vi "testLeonardo.vi"() -> ()   [LabVIEW 2014]
panel:
  out "Buttons":bool[](array[boolean])
  in  "stop":bool
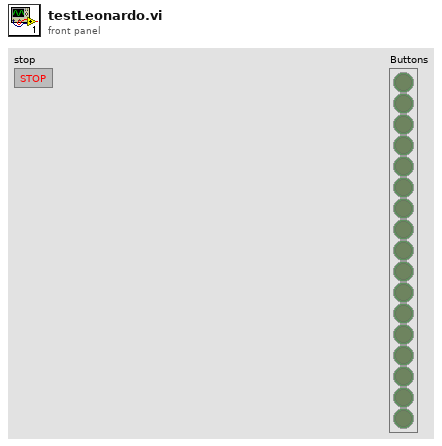
[diagram p1: front panel]
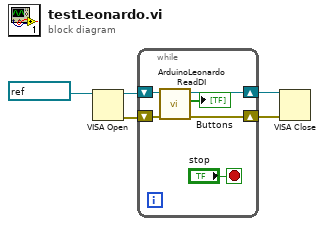
[diagram p0: block diagram]
diagram:
  n1 = VISA Open(VISA resource name=refnum<visa-resource-name> "COM4") -> (VISA resource name=w5:refnum<visa-resource-name>, error out=w1:errorcluster)  [unwired: 4 in]
  n2 = while {
    shift-right: [w9] -> w2
    shift-left: w5 -> [w11]
    shift-right: [w10] -> w3
    shift-left: w1 -> [w8]
    stop <- "stop" stop-if-true
    n3 = call "ArduinoLeonardoReadDI.vi"("error in (no error)"=w8, "VISA resource name"=w11) -> ("error out"=w10:errorcluster, "Buttons"=→"Buttons":bool[], "VISA resource name out"=w9:refnum<visa-resource-name>)  [unwired: 7 in]
  }
  n4 = VISA Close(VISA resource name=w2, error in (no error)=w3) -> ()  [unwired: 1 out]
